vi "Get Image Info.vi"(7 "Note Type IN":T2={"TDI Actions"=enum."Set Height", "Width (X)"=[], "Cmd Received?"=FALSE, "Display Height (Y)"=1, "Acquisition Line Rate"=8000.0, "Pixel format"=257, "Binning Horizontal (X)"=1, "Binning Vertical (Y)"=1, "Scan Direction"=0, "TDI Stages"=256, "Reverse X"=FALSE, "Test Pattern"=0, "Running?"=FALSE, "Image Reference"=refnum, "Number of frames"=1, "Segments per Buffer"=1, "Recorded Height"=1, "Display Binning Factor"=1, "File Path"=path ""} {"Display Binning Factor" min=1; "Test Pattern" items=["Off", "Grey Horizontal Ramp", "Grey Diagonal Ramp", "Grey Diagonal Ramp Moving"]; "TDI Stages" items=["4"=4, "8"=8, "16"=16, "32"=32, "64"=64, "96"=96, "128"=128, "160"=160, "192"=192, "224"=224, "240"=240, "248"=248, "252"=252, "256"=256]; "Scan Direction" items=["Forward", "Reverse", "LineIn"]; "Binning Vertical (Y)" items=["X1"=1, "X2"=2, "X4"=4, "X8"=8]; "Binning Horizontal (X)" items=["X1"=1, "X2"=2, "X4"=4, "X8"=8]; "Pixel format" items=["Mono8"=257, "Mono10"=258, "Mono12"=259]}) -> (8 "output cluster":T1={"Image Width (Pixels)"=0, "Image Height (Pixels)"=0, "Pixel Width (µm)"=1.0, "Pixel Height (µm)"=1.0, "Bits Per Sample (e.g. 16)"=0, "No. of Frames"=0, "No. of Slices"=0, "Time Step (sec)"=0.0, "Z Step (µm)"=0.0})   [LabVIEW 2020]
uses:
  VPD Controls/VPD Note Type.ctl
  VPD Controls/VPD Actions.ctl
  VPD Controls/VPD Pixel format.ctl
  VPD Controls/VPD Binning XX.ctl
  VPD Controls/VPD Scan Direction.ctl
  VPD Controls/VPD TDI Stages.ctl
  VPD Controls/VPD Test Pattern.ctl
  <vilib>/vision/Image Controls.llb/IMAQ Image.ctl
  Tools/TIFF Image Read and Write/ImageJ TIF Type Defs/TIF Write Image Information.ctl
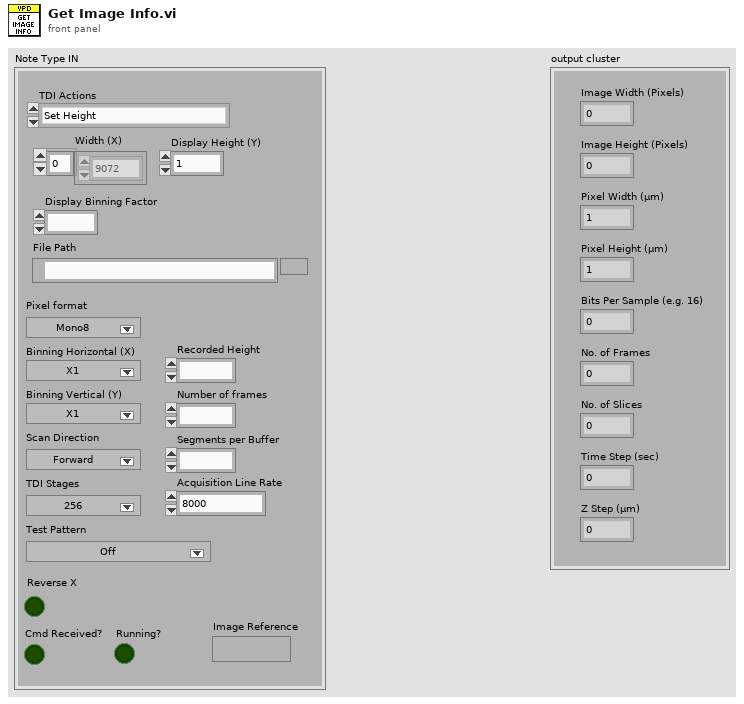
[diagram p1: front panel]
types:
  T1 = typedef "TIF Write Image Information.ctl" = cluster{"Image Width (Pixels)":u32, "Image Height (Pixels)":u32, "Pixel Width (µm)":dbl, "Pixel Height (µm)":dbl, "Bits Per Sample (e.g. 16)":u32, "No. of Frames":u32, "No. of Slices":u32, "Time Step (sec)":dbl, "Z Step (µm)":dbl}
  T2 = typedef "VPD Note Type.ctl" = cluster{"TDI Actions":T3, "Width (X)":i64[], "Cmd Received?":bool, "Display Height (Y)":i64, "Acquisition Line Rate":dbl, "Pixel format":T4, "Binning Horizontal (X)":T5, "Binning Vertical (Y)":T5, "Scan Direction":T6, "TDI Stages":T7, "Reverse X":bool, "Test Pattern":T8, "Running?":bool, "Image Reference":T9, "Number of frames":i32, "Segments per Buffer":i64, "Recorded Height":u32, "Display Binning Factor":i32, "File Path":path}
  T3 = typedef "VPD Actions.ctl" = enum16{"Nothing", "Set Height", "Set ROI", "Set Pixel format", "Set Line rate", "Set Binning Horizontal", "Set Binning Vertical", "Set Scan Direction", "Set TDI Stages", "Set Reverse X", "Set Test Pattern", "Set Segments per Buffer", "Set Display Binning Factor", "Live", "Record", "Quit"}
  T4 = typedef "VPD Pixel format.ctl" = i64
  T5 = typedef "VPD Binning XX.ctl" = u16
  T6 = typedef "VPD Scan Direction.ctl" = i64
  T7 = typedef "VPD TDI Stages.ctl" = u16
  T8 = typedef "VPD Test Pattern.ctl" = u16
  T9 = typedef "IMAQ Image.ctl" = refnum<image>
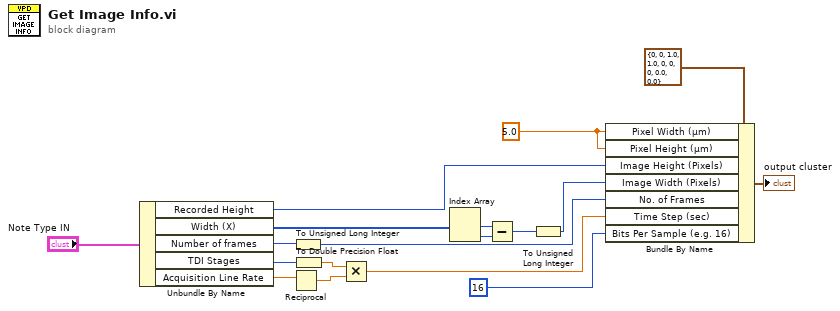
[diagram p0: block diagram]
diagram:
  w2 = 5.0
  n1 = Unbundle By Name("Note Type IN") -> ("Recorded Height"=w3:u32, "Width (X)"=w8:i64[], "Number of frames"=w10:i32, "TDI Stages"=w12:T7, "Acquisition Line Rate"=w13:dbl)
  n2 = Reciprocal(x=w13) -> (1/x=w16:dbl)
  n3 = To Unsigned Long Integer(number=w10) -> (unsigned 32bit integer=w9:u32)
  n4 = To Double Precision Float(number=w12) -> (double precision float=w15:dbl)
  n5 = Multiply(x=w15, y=w16) -> (x*y=w11:dbl)
  n6 = Index Array(array=w8) -> (element #1=w6:i64, element #2=w7:i64)  [unwired: 2 in]
  n7 = Subtract(x=w6, y=w7) -> (x-y=w5:i64)
  n8 = To Unsigned Long Integer(number=w5) -> (unsigned 32bit integer=w4:u32)
  n9 = Bundle By Name(cluster=T1 {"Image Width (Pixels)"=0, "Image Height (Pixels)"=0, "Pixel Width (µm)"=1.0, "Pixel Height (µm)"=1.0, "Bits Per Sample (e.g. 16)"=0, "No. of Frames"=0, "No. of Slices"=0, "Time Step (sec)"=0.0, "Z Step (µm)"=0.0} ("Image Info"), "Pixel Width (µm)"=w2, "Pixel Height (µm)"=w2, "Image Height (Pixels)"=w3, "Image Width (Pixels)"=w4, "No. of Frames"=w9, "Time Step (sec)"=w11, "Bits Per Sample (e.g. 16)"=u32 16) -> (→"output cluster":T1)
